vi "3 Totes Forward.vi"   [LabVIEW 2014]
types:
  T1 = enum16{"Move Forward", "Move Backward", "Strafe Right", "Strafe Left"}
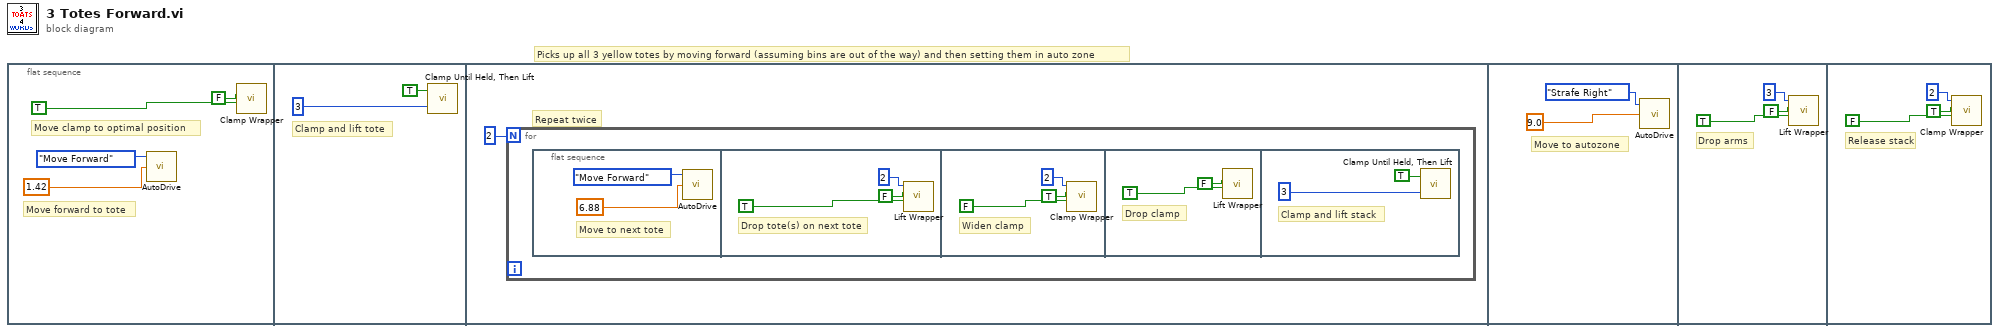
[diagram p0: block diagram]
diagram:
  # "Picks up all 3 yellow totes by moving forward (assuming bins are out of the way) and then setting them in auto zone"
  n1 = flat-sequence {
    frame #0 {
      # "Move clamp to optimal position"
      # "Move forward to tote"
      n2 = call "AutoDrive.vi"("Distance (ft)"=1.42 ("Feet"), "Direction"=T1."Move Forward") -> ()  [unwired: 1 in, 1 out]
      n3 = call "Clamp Wrapper.vi"("In"=TRUE, "Out"=FALSE) -> ()  [unwired: 2 in]
    }
    frame #1 {
      # "Clamp and lift tote"
      n4 = call "Clamp Until Held, Then Lift.vi"("Iterations"=3, "Clamp + Lift"=TRUE) -> ()  [unwired: 1 in]
    }
    frame #2 {
      # "Repeat twice"
      n5 = for {
        N: 2 -> [_]
        n6 = flat-sequence {
          frame #0 {
            # "Move to next tote"
            n7 = call "AutoDrive.vi"("Distance (ft)"=6.88 ("Feet"), "Direction"=T1."Move Forward") -> ()  [unwired: 1 in, 1 out]
          }
          frame #1 {
            # "Drop tote(s) on next tote"
            n8 = call "Lift Wrapper.vi"("Down"=TRUE, "Up"=FALSE, "Iterations"=2) -> ()  [unwired: 1 in]
          }
          frame #2 {
            # "Widen clamp"
            n9 = call "Clamp Wrapper.vi"("In"=FALSE ("In or Out"), "Out"=TRUE, "Iterations"=2) -> ()  [unwired: 1 in]
          }
          frame #3 {
            # "Drop clamp"
            n10 = call "Lift Wrapper.vi"("Down"=TRUE ("Up or Down"), "Up"=FALSE) -> ()  [unwired: 2 in]
          }
          frame #4 {
            # "Clamp and lift stack"
            n11 = call "Clamp Until Held, Then Lift.vi"("Iterations"=3, "Clamp + Lift"=TRUE) -> ()  [unwired: 1 in]
          }
        }
      }
    }
    frame #3 {
      # "Move to autozone"
      n12 = call "AutoDrive.vi"("Distance (ft)"=9.0 ("Feet"), "Direction"=T1."Strafe Right") -> ()  [unwired: 1 in, 1 out]
    }
    frame #4 {
      # "Drop arms"
      n13 = call "Lift Wrapper.vi"("Down"=TRUE ("Up or Down"), "Up"=FALSE, "Iterations"=3) -> ()  [unwired: 1 in]
    }
    frame #5 {
      # "Release stack"
      n14 = call "Clamp Wrapper.vi"("In"=FALSE ("In or Out"), "Out"=TRUE, "Iterations"=2) -> ()  [unwired: 1 in]
    }
  }
